vi "Kill Service.vi"(8 "error in":errorcluster, 11 "full exe name":string) -> (0 "error out":errorcluster)   [LabVIEW 2020, in "MeasurementServerTests.lvlib"]
uses:
  MeasurementServerTests.lvlib
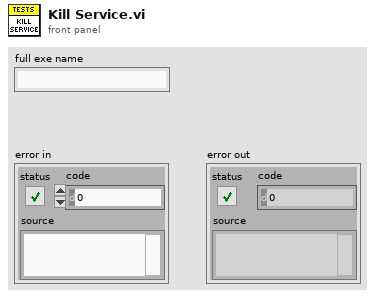
[diagram p1: front panel]
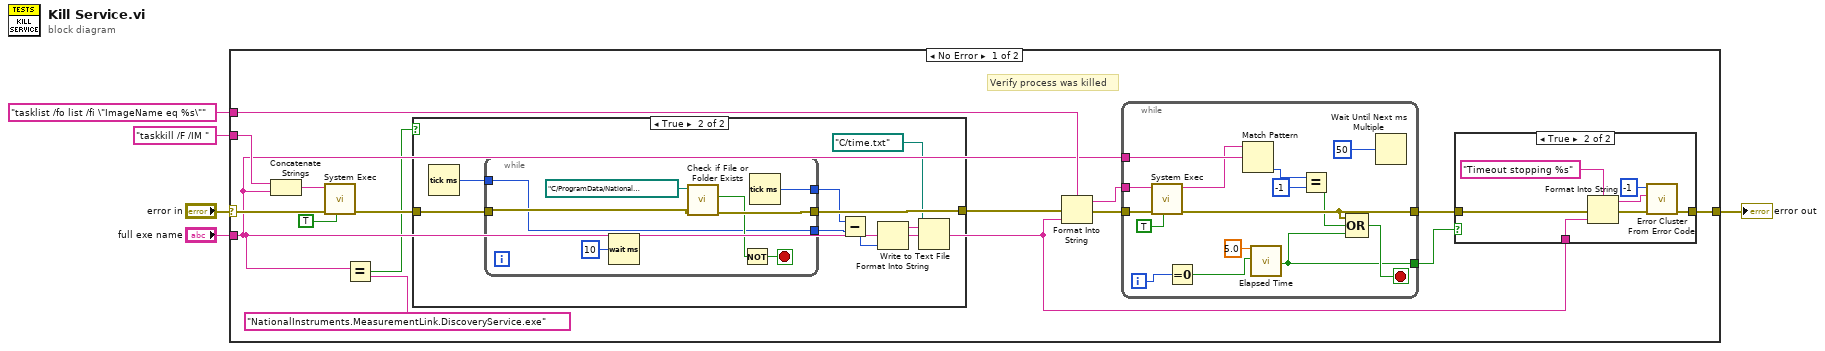
[diagram p0: block diagram]
diagram:
  n1 = case shown="No Error" "error in" {
    selector: "error in" -> [w14 w61]
    tunnel: "taskkill /F /IM " -> [w20 _]
    tunnel: "tasklist /fo list /fi \"ImageName eq %s\"" -> [w16 _]
    tunnel: "full exe name" -> [w7 _]
    tunnel: [w11 w61] -> w1
    frame No Error {
      # "Verify process was killed"
      n2 = Concatenate Strings(w20, w7) -> (w19:string)
      n3 = call <vilib>:"System Exec.vi"("run minimized? (F)"=TRUE, "error in (no error)"=w14, "command line"=w19) -> ("error out"=w10:errorcluster)  [unwired: 5 in, 3 out]
      n4 = Equal?(x=w7, y="NationalInstruments.MeasurementLink.DiscoveryService.exe") -> (x = y?=w6:bool)
      n5 = case shown="True" w6 {
        tunnel: w10 -> [w21 w29]
        tunnel: [w21 w28] -> w9
        frame False {
        }
        frame True {
          n6 = Tick Count (ms)() -> (millisecond timer value=w27:u32)
          n7 = while {
            tunnel: w29 -> [w37]
            tunnel: [w36] -> w28
            tunnel: w27 -> [w31]
            tunnel: [w32] -> w26
            tunnel: [w31] -> w25
            stop <- w35 stop-if-true
            n8 = Wait (ms)(milliseconds to wait=u32 10) -> ()  [unwired: 1 out]
            n9 = call <vilib>:"Check if File or Folder Exists.vi"("error in (no error)"=w37, "path"=path "C:/ProgramData/National Instruments/MeasurementLink/Discovery/v1/DiscoveryService.json") -> ("error out"=w36:errorcluster, "file or folder exists?"=w34:bool)  [unwired: 7 in, 1 out]
            n10 = Not(x=w34) -> (.not. x?=w35:bool)
            n11 = Tick Count (ms)() -> (millisecond timer value=w32:u32)
          }
          n12 = Subtract(x=w26, y=w25) -> (x-y=w24:u32)
          n13 = Format Into String(w24) -> (resulting string=w23:string)  [unwired: 3 in, 1 out]
          n14 = Write to Text File(file (use dialog)=path "C:/time.txt", text=w23) -> ()  [unwired: 2 in, 3 out]
        }
      }
      n15 = Format Into String(format string=w16, error in=w9, w7) -> (resulting string=w15:string, error out=w17:errorcluster)  [unwired: 1 in]
      n16 = while {
        tunnel: w7 -> [w59]
        tunnel: w15 -> [w56]
        tunnel: w17 -> [w60]
        tunnel: [w52] -> w13
        tunnel: [w48] -> w12
        i -> [w47]
        stop <- w50 stop-if-true
        n17 = call <vilib>:"System Exec.vi"("run minimized? (F)"=TRUE, "error in (no error)"=w60, "command line"=w56) -> ("error out"=w52:errorcluster, "standard output"=w55:string)  [unwired: 5 in, 2 out]
        n18 = Equal To 0?(x=w47) -> (x = 0?=w46:bool)
        n19 = Match Pattern(string=w55, regular expression=w59) -> (offset past match=w58:i32)  [unwired: 1 in, 3 out]
        n20 = call "Elapsed Time"("Time Target (s)"=5.0, "Reset"=w46) -> ("Time has Elapsed"=w48:bool)  [unwired: 10 in, 7 out]
        n21 = Equal?(x=w58, y=-1) -> (x = y?=w51:bool)
        n22 = Compound Arithmetic op=OR(w52, w51, w48) -> (w50:bool)
        n23 = Wait Until Next ms Multiple(millisecond multiple=u32 50) -> ()  [unwired: 1 out]
      }
      n24 = case shown="True" w12 {
        tunnel: w13 -> [w38 w43]
        tunnel: [w38 w45] -> w11
        tunnel: w7 -> [_ w41]
        frame False {
        }
        frame True {
          n25 = Format Into String(format string="Timeout stopping %s", error in=w43, w41) -> (resulting string=w39:string, error out=w42:errorcluster)  [unwired: 1 in]
          n26 = call <vilib>:"Error Cluster From Error Code.vi"("error in (no error)"=w42, "error message (\"\")"=w39, "error code (0)"=-1) -> ("error out"=w45:errorcluster)  [unwired: 6 in]
        }
      }
    }
    frame Error {
    }
  }
  "error out" <- w1
